vi "8846.vi"() -> ()   [LabVIEW 2014]
doc: "This example shows how to configure a measurement and take a single reading."
uses:
  <vilib>/Utility/error.llb/DialogType.ctl
  8846/Fluke 884X Series/Public/Data/Read (Single Point).vi
  <vilib>/httpClient/POSTBuffer.vi
  8846/Fluke 884X Series/Fluke 884X Series.lvlib
  <vilib>/httpClient/LabVIEWHTTPClient.lvlib
panel:
  in  "字符串":string
  out "已用时间":string
  out "平均值":dbl
  out "最小值":dbl
  out "最大值":dbl
  in  "测试项目":u16(ring)=4 items=["DC Voltage", "AC Voltage", "2 - Wire Resistance", "4 - Wire Resistance", "DC Current", "AC Current", "Frequency", "Period", "Continuity", "Diode Checking", "Temperature", "Capacitance"]
  in  "停止":bool
  out "电压/电流":dbl[](graph)
  out "实时测量数值":dbl
  in  "串口":refnum<visa-resource-name>
  # "FLUKE 8846A台式万用表静电流采集V2.0"
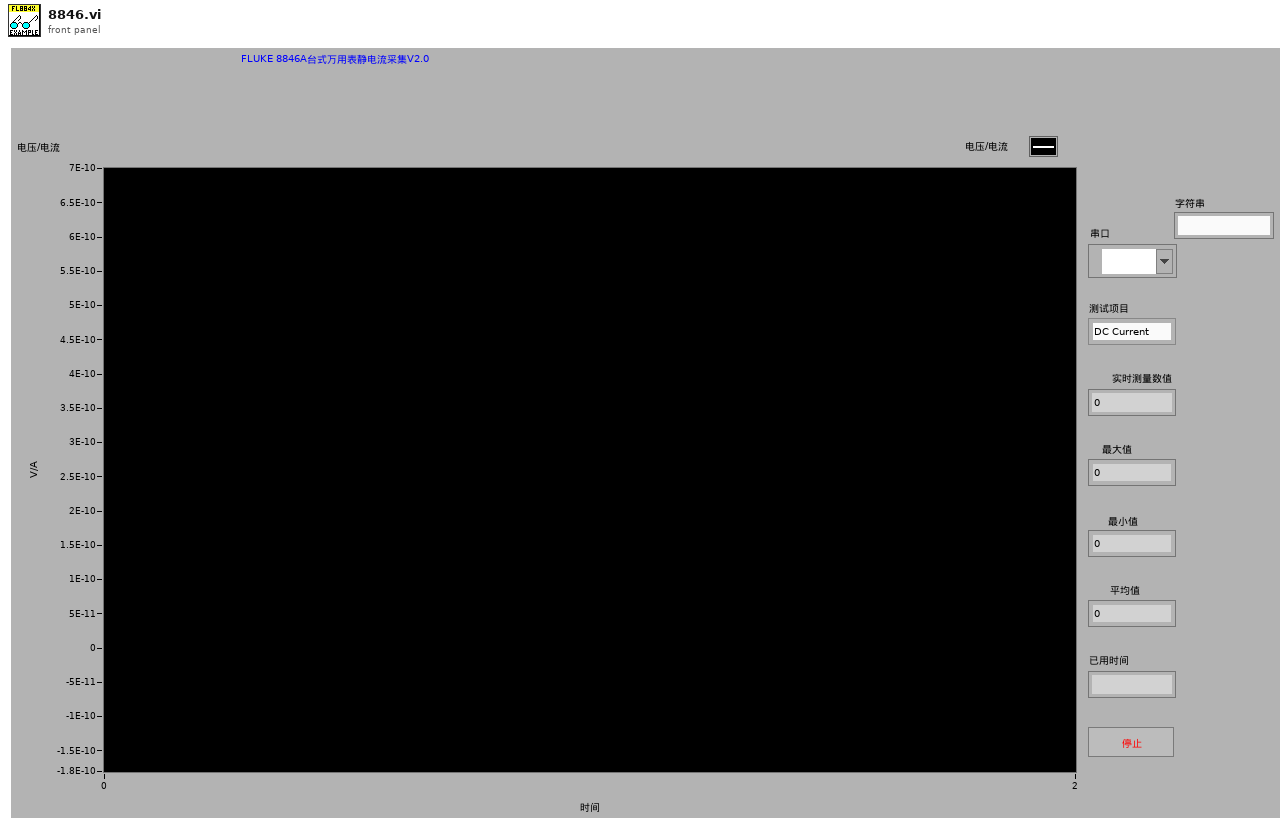
[diagram p1: front panel]
types:
  T1 = cluster{"Baud Rate":u32, "Parity":u16, "Data Bits":u16, "Stop Bits":u16, "Flow Control":u16}
  T2 = enum16{"None", "Min/Max", "Null", "dB", "dBm", "Limit"}
  T3 = typedef "DialogType.ctl" = u16
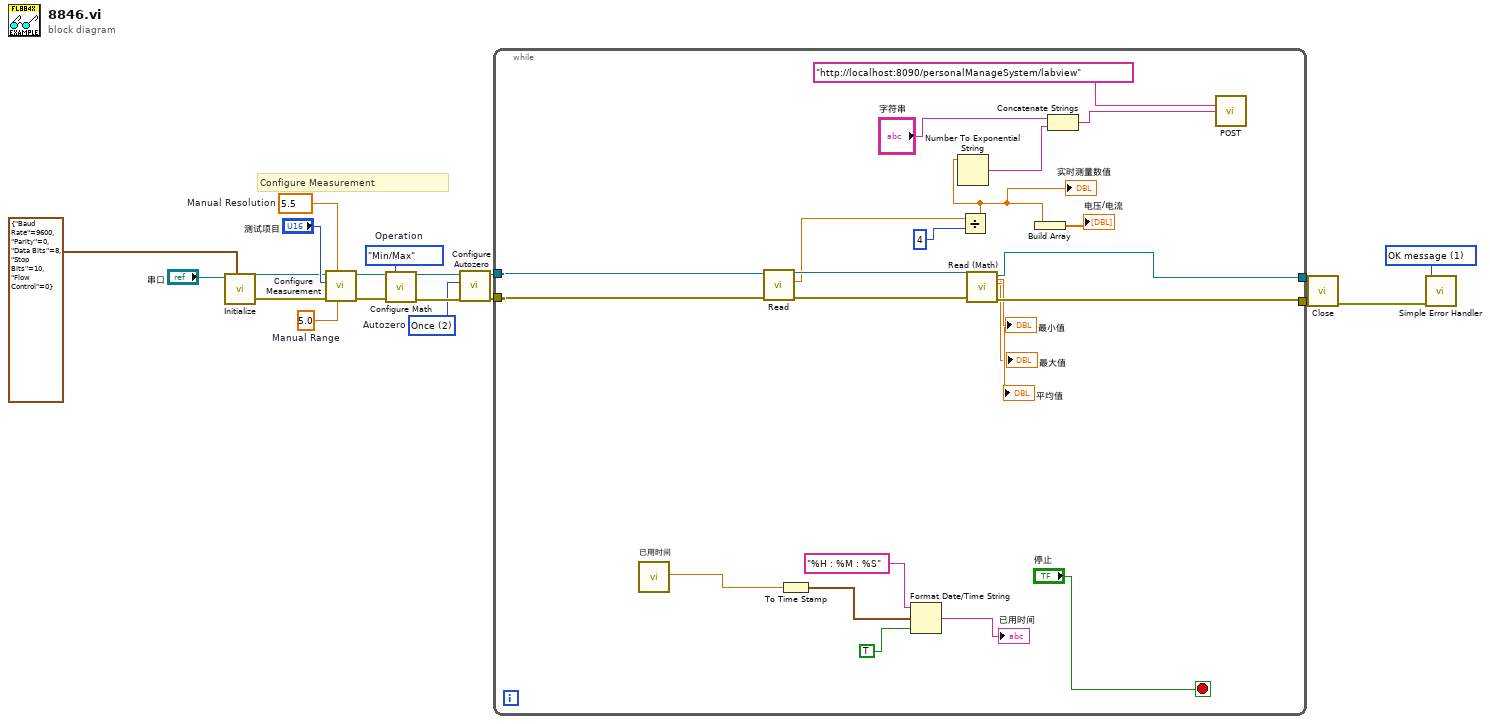
[diagram p0: block diagram]
diagram:
  w6 = 5.0  # Manual Range
  w7 = 5.5 items=["4.5"=4.5, "5.5"=5.5, "6.5"=6.5]  # Manual Resolution
  w8 = u16 2 items=["On", "Off", "Once"]  # Autozero
  w9 = T2."Min/Max"  # Operation
  w18 = T3 1 items=["no dialog", "OK message", "continue or stop message", "OK message + warnings", "continue/stop + warnings"] ("type of dialog (OK msg:1)")
  # "Configure Measurement"
  n1 = call "Initialize.vi"("Serial Configuration"=T1 {"Baud Rate"=9600, "Parity"=0, "Data Bits"=8, "Stop Bits"=10, "Flow Control"=0}, "VISA resource name"="串口") -> ("error out"=w4:errorcluster, "VISA resource name out"=w5:refnum<visa-resource-name>)  [unwired: 8 in]
  n2 = call "Configure Measurement.vi"("Manual Range (1.0)"=w6, "Manual Resolution (5.5 Digits)"=w7, "error in (no error)"=w4, "Function (0: DC Voltage)"="测试项目", "VISA resource name"=w5) -> ("error out"=w13:errorcluster, "VISA resource name out"=w14:refnum<visa-resource-name>)  [unwired: 5 in]
  n3 = call "Configure Math.vi"("VISA resource name"=w14, "Operation (0:None)"=w9, "error in (no error)"=w13) -> ("VISA resource name out"=w12:refnum<visa-resource-name>, "error out"=w11:errorcluster)  [unwired: 11 in]
  n4 = call "Configure Autozero.vi"("error in (no error)"=w11, "Autozero  (0: On)"=w8, "VISA resource name"=w12) -> ("error out"=w2:errorcluster, "VISA resource name out"=w3:refnum<visa-resource-name>)  [unwired: 7 in]
  n5 = while {
    tunnel: [w37] -> w16
    tunnel: [w35] -> w15
    tunnel: w3 -> [w38]
    tunnel: w2 -> [w36]
    stop <- "停止" stop-if-true
    n6 = call "已用时间"() -> ("Elapsed Time (s)"=w34:dbl)  [unwired: 12 in, 7 out]
    n7 = call-poly "Read.vi"("error in (no error)"=w36, "VISA resource name"=w38) -> ("error out"=w28:errorcluster, "Measurement"=w26:dbl, "VISA resource name out"=w29:refnum<visa-resource-name>)  [unwired: 7 in]
    n8 = To Time Stamp(1:w34) -> (0:w42:timestamp)
    n9 = Format Date/Time String(time format string (%c)="%H : %M : %S", seconds (now)=w42, UTC format=TRUE) -> (date/time string=→"已用时间":string)
    n10 = Divide(x=w26, y=4) -> (x/y=w23:dbl)
    "实时测量数值" <- w23
    n11 = Number To Exponential String(number=w23) -> (E-format string=w20:string)  [unwired: 3 in]
    n12 = call "Read (Math).vi"("error in (no error)"=w28, "VISA resource name"=w29) -> ("error out"=w35:errorcluster, "Average"=→"平均值":dbl, "VISA resource name out"=w37:refnum<visa-resource-name>, "Minimum"=→"最小值":dbl, "Maximum"=→"最大值":dbl)  [unwired: 4 in, 1 out]
    n13 = Build Array(w23) -> (→"电压/电流":dbl[])
    n14 = Concatenate Strings("字符串", w20) -> (w22:string)
    n15 = call-poly <vilib>:"POST.vi"("url"="http://localhost:8090/personalManageSystem/labview", "buffer"=w22) -> ()  [unwired: 10 in, 4 out]
  }
  n16 = call "Close.vi"("error in (no error)"=w15, "VISA resource name"=w16) -> ("error out"=w19:errorcluster)  [unwired: 9 in]
  n17 = call <vilib>:"Simple Error Handler.vi"("type of dialog (OK msg:1)"=w18, "error in (no error)"=w19) -> ()  [unwired: 3 in, 5 out]
